vi "VI Tree.vi"   [LabVIEW 2014, in "Newport ESP301.lvlib"]
doc: "This is the instrument driver for the <INSTRUMENT NAME>. The VI Tree displays all the user-callable VIs of the instrument driver in an organized table.\n\nNOTE :\nEvery VIs need the VISA Ressource Name parameter for working."
uses:
  Newport ESP301.lvlib
panel:
  # "(c) 2009 <Newport>.  ALL RIGHTS RESERVED."
  # "SEE DIAGRAM\nFOR VI TREE."
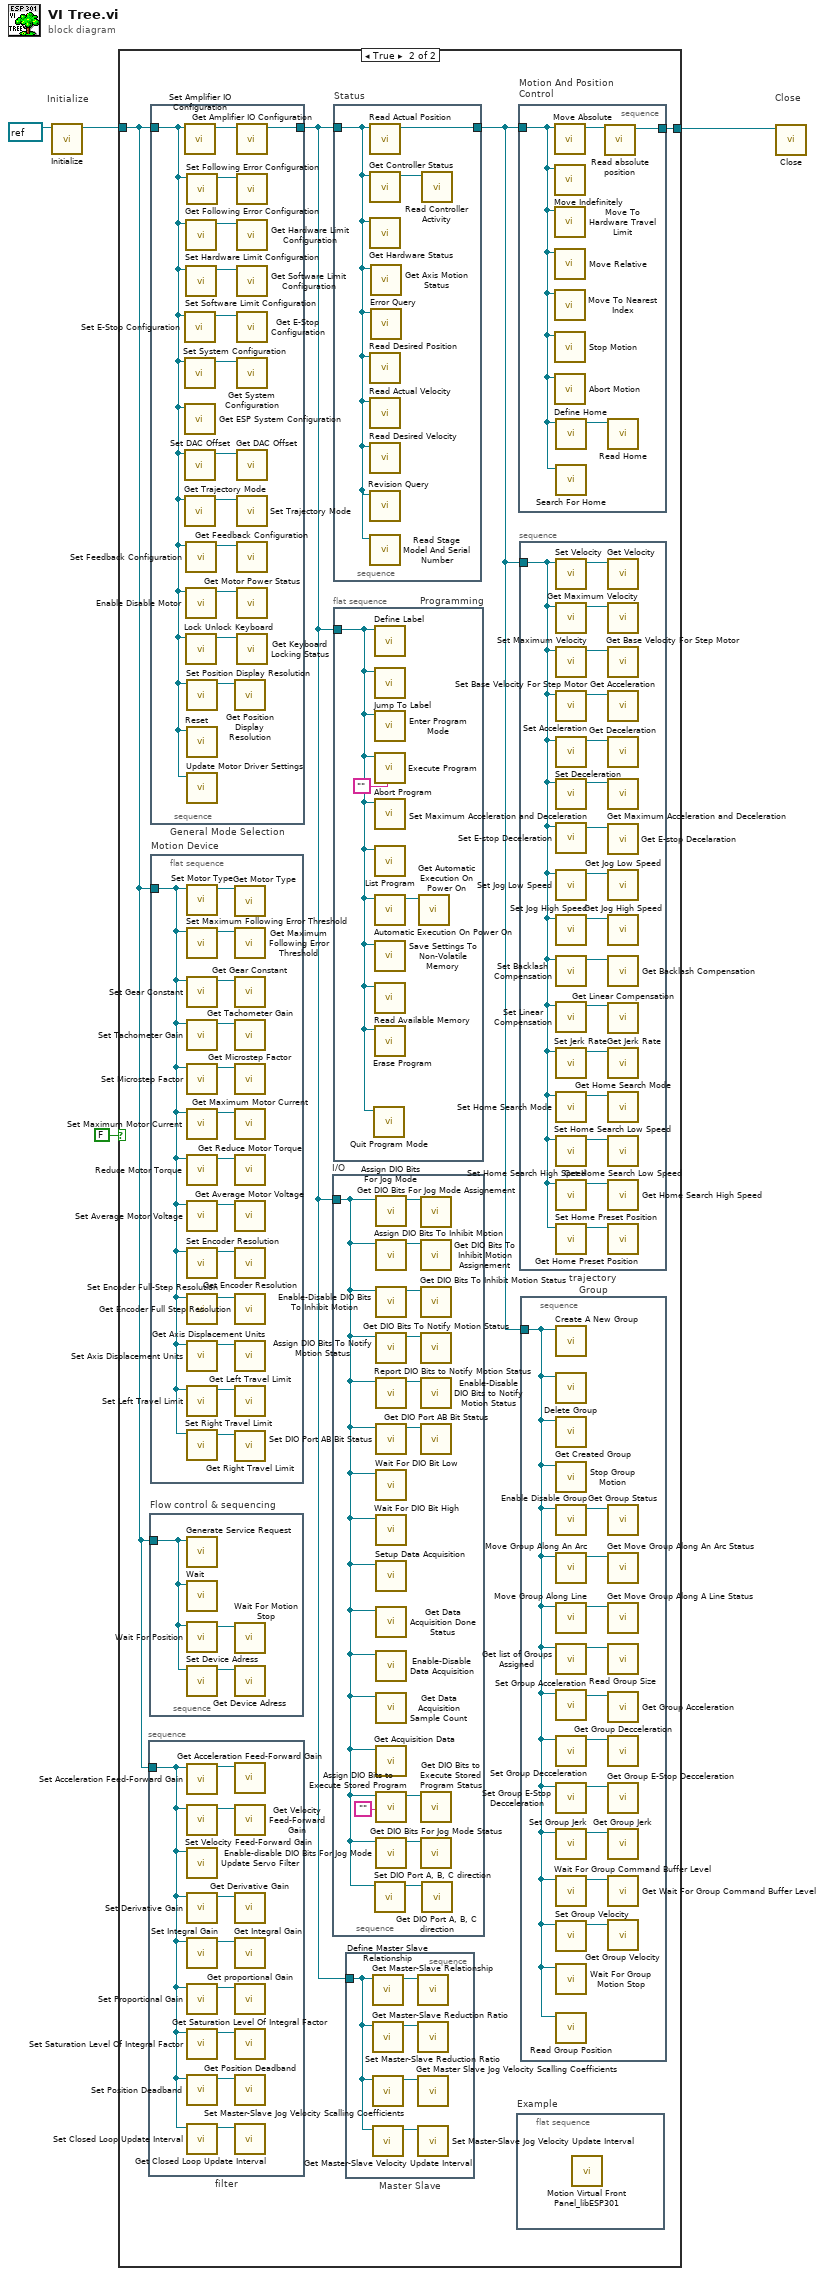
[diagram p0: block diagram]
diagram:
  # "Close"
  # "Initialize"
  n1 = call "Initialize.vi"("VISA resource name"=refnum<visa-resource-name> refnum) -> ("VISA resource name out"=w3:refnum<visa-resource-name>)  [unwired: 8 in, 1 out]
  n2 = case shown="True" FALSE {
    tunnel: w3 -> [w5 w8]
    tunnel: [w5 w6] -> w2
    frame False {
    }
    frame True {
      n3 = stacked-sequence "filter" {
        tunnel: w8 -> [w65]
        frame #0 {
          n4 = call "Set Acceleration Feed-Forward Gain.vi"("VISA resource name"=w65) -> ("VISA resource name out"=w66:refnum<visa-resource-name>)  [unwired: 5 in, 1 out]
          n5 = call "Set Velocity Feed-Forward Gain.vi"("VISA resource name"=w65) -> ("VISA resource name out"=w67:refnum<visa-resource-name>)  [unwired: 5 in, 1 out]
          n6 = call "Update Servo Filter.vi"("VISA resource name"=w65) -> ()  [unwired: 5 in, 2 out]
          n7 = call "Set Derivative Gain.vi"("VISA resource name"=w65) -> ("VISA resource name out"=w71:refnum<visa-resource-name>)  [unwired: 5 in, 1 out]
          n8 = call "Set Integral Gain.vi"("VISA resource name"=w65) -> ("VISA resource name out"=w72:refnum<visa-resource-name>)  [unwired: 5 in, 1 out]
          n9 = call "Set Proportional Gain.vi"("VISA resource name"=w65) -> ("VISA resource name out"=w70:refnum<visa-resource-name>)  [unwired: 5 in, 1 out]
          n10 = call "Set Saturation Level Of Integral Factor.vi"("VISA resource name"=w65) -> ("VISA resource name out"=w69:refnum<visa-resource-name>)  [unwired: 5 in, 1 out]
          n11 = call "Set Position Deadband.vi"("VISA resource name"=w65) -> ("VISA resource name out"=w68:refnum<visa-resource-name>)  [unwired: 5 in, 1 out]
          n12 = call "Set Closed Loop Update Interval.vi"("VISA resource name"=w65) -> ("VISA resource name out"=w64:refnum<visa-resource-name>)  [unwired: 5 in, 1 out]
          n13 = call "Get Acceleration Feed-Forward Gain.vi"("VISA resource name"=w66) -> ()  [unwired: 4 in, 3 out]
          n14 = call "Get Velocity Feed-Forward Gain.vi"("VISA resource name"=w67) -> ()  [unwired: 4 in, 3 out]
          n15 = call "Get Derivative Gain.vi"("VISA resource name"=w71) -> ()  [unwired: 4 in, 3 out]
          n16 = call "Get Integral Gain.vi"("VISA resource name"=w72) -> ()  [unwired: 4 in, 3 out]
          n17 = call "Get proportional Gain.vi"("VISA resource name"=w70) -> ()  [unwired: 4 in, 3 out]
          n18 = call "Get Saturation Level Of Integral Factor.vi"("VISA resource name"=w69) -> ()  [unwired: 4 in, 3 out]
          n19 = call "Get Position Deadband.vi"("VISA resource name"=w68) -> ()  [unwired: 4 in, 3 out]
          n20 = call "Get Closed Loop Update Interval.vi"("VISA resource name"=w64) -> ()  [unwired: 4 in, 3 out]
        }
      }
      n21 = stacked-sequence "Flow control & sequencing" {
        tunnel: w8 -> [w36]
        frame #0 {
          n22 = call "Generate Service Request.vi"("VISA resource name"=w36) -> ()  [unwired: 5 in, 2 out]
          n23 = call "Wait.vi"("VISA resource name"=w36) -> ()  [unwired: 5 in, 2 out]
          n24 = call "Wait For Position.vi"("VISA resource name"=w36) -> ("VISA resource name out"=w38:refnum<visa-resource-name>)  [unwired: 5 in, 1 out]
          n25 = call "Set Device Adress.vi"("VISA resource name"=w36) -> ("VISA resource name out"=w37:refnum<visa-resource-name>)  [unwired: 5 in, 1 out]
          n26 = call "Wait For Motion Stop.vi"("VISA resource name"=w38) -> ()  [unwired: 5 in, 2 out]
          n27 = call "Get Device Adress.vi"("VISA resource name"=w37) -> ()  [unwired: 4 in, 3 out]
        }
      }
      n28 = stacked-sequence "General Mode Selection" {
        tunnel: w8 -> [w23]
        tunnel: [w22] -> w7
        frame #0 {
          n29 = call "Set Amplifier IO Configuration.vi"("VISA resource name"=w23) -> ("VISA resource name out"=w31:refnum<visa-resource-name>)  [unwired: 5 in, 1 out]
          n30 = call "Set E-Stop Configuration.vi"("VISA resource name"=w23) -> ("VISA resource name out"=w32:refnum<visa-resource-name>)  [unwired: 5 in, 1 out]
          n31 = call "Set System Configuration.vi"("VISA resource name"=w23) -> ("VISA resource name out"=w28:refnum<visa-resource-name>)  [unwired: 5 in, 1 out]
          n32 = call "Get ESP System Configuration.vi"("VISA resource name"=w23) -> ()  [unwired: 4 in, 3 out]
          n33 = call "Set DAC Offset.vi"("VISA resource name"=w23) -> ("VISA resource name out"=w30:refnum<visa-resource-name>)  [unwired: 5 in, 1 out]
          n34 = call "Get Trajectory Mode.vi"("VISA resource name"=w23) -> ("VISA resource name out"=w29:refnum<visa-resource-name>)  [unwired: 4 in, 2 out]
          n35 = call "Set Hardware Limit Configuration.vi"("VISA resource name"=w23) -> ("VISA resource name out"=w35:refnum<visa-resource-name>)  [unwired: 5 in, 1 out]
          n36 = call "Set Software Limit Configuration.vi"("VISA resource name"=w23) -> ("VISA resource name out"=w33:refnum<visa-resource-name>)  [unwired: 5 in, 1 out]
          n37 = call "Set Feedback Configuration.vi"("VISA resource name"=w23) -> ("VISA resource name out"=w27:refnum<visa-resource-name>)  [unwired: 5 in, 1 out]
          n38 = call "Enable Disable Motor.vi"("VISA resource name"=w23) -> ("VISA resource name out"=w26:refnum<visa-resource-name>)  [unwired: 5 in, 1 out]
          n39 = call "Lock Unlock Keyboard.vi"("VISA resource name"=w23) -> ("VISA resource name out"=w25:refnum<visa-resource-name>)  [unwired: 5 in, 1 out]
          n40 = call "Set Following Error Configuration.vi"("VISA resource name"=w23) -> ("VISA resource name out"=w34:refnum<visa-resource-name>)  [unwired: 5 in, 1 out]
          n41 = call "Set Position Display Resolution.vi"("VISA resource name"=w23) -> ("VISA resource name out"=w24:refnum<visa-resource-name>)  [unwired: 5 in, 1 out]
          n42 = call "Reset.vi"("VISA resource name"=w23) -> ()  [unwired: 5 in, 2 out]
          n43 = call "Update Motor Driver Settings.vi"("VISA resource name"=w23) -> ()  [unwired: 5 in, 2 out]
          n44 = call "Get Position Display Resolution.vi"("VISA resource name"=w24) -> ()  [unwired: 4 in, 3 out]
          n45 = call "Get Amplifier IO Configuration.vi"("VISA resource name"=w31) -> ("VISA resource name out"=w22:refnum<visa-resource-name>)  [unwired: 4 in, 2 out]
          n46 = call "Get Following Error Configuration.vi"("VISA resource name"=w34) -> ()  [unwired: 4 in, 3 out]
          n47 = call "Get Hardware Limit Configuration.vi"("VISA resource name"=w35) -> ()  [unwired: 4 in, 3 out]
          n48 = call "Get Software Limit Configuration.vi"("VISA resource name"=w33) -> ()  [unwired: 4 in, 3 out]
          n49 = call "Get E-Stop Configuration.vi"("VISA resource name"=w32) -> ()  [unwired: 4 in, 3 out]
          n50 = call "Get System Configuration.vi"("VISA resource name"=w28) -> ()  [unwired: 4 in, 3 out]
          n51 = call "Get DAC Offset.vi"("VISA resource name"=w30) -> ()  [unwired: 4 in, 3 out]
          n52 = call "Set Trajectory Mode.vi"("VISA resource name"=w29) -> ()  [unwired: 6 in, 2 out]
          n53 = call "Get Feedback Configuration.vi"("VISA resource name"=w27) -> ()  [unwired: 4 in, 3 out]
          n54 = call "Get Motor Power Status.vi"("VISA resource name"=w26) -> ()  [unwired: 4 in, 3 out]
          n55 = call "Get Keyboard Locking Status.vi"("VISA resource name"=w25) -> ()  [unwired: 4 in, 3 out]
        }
      }
      n56 = flat-sequence "Motion Device" {
        tunnel: w8 -> [w91]
        frame #0 {
          n57 = call "Set Motor Type.vi"("VISA resource name"=w91) -> ("VISA resource name out"=w103:refnum<visa-resource-name>)  [unwired: 6 in, 1 out]
          n58 = call "Set Maximum Following Error Threshold.vi"("VISA resource name"=w91) -> ("VISA resource name out"=w102:refnum<visa-resource-name>)  [unwired: 5 in, 1 out]
          n59 = call "Set Gear Constant.vi"("VISA resource name"=w91) -> ("VISA resource name out"=w99:refnum<visa-resource-name>)  [unwired: 5 in, 1 out]
          n60 = call "Set Tachometer Gain.vi"("VISA resource name"=w91) -> ("VISA resource name out"=w101:refnum<visa-resource-name>)  [unwired: 5 in, 1 out]
          n61 = call "Set Microstep Factor.vi"("VISA resource name"=w91) -> ("VISA resource name out"=w100:refnum<visa-resource-name>)  [unwired: 5 in, 1 out]
          n62 = call "Set Maximum Motor Current.vi"("VISA resource name"=w91) -> ("VISA resource name out"=w90:refnum<visa-resource-name>)  [unwired: 5 in, 1 out]
          n63 = call "Reduce Motor Torque.vi"("VISA resource name"=w91) -> ("VISA resource name out"=w98:refnum<visa-resource-name>)  [unwired: 6 in, 1 out]
          n64 = call "Set Average Motor Voltage.vi"("VISA resource name"=w91) -> ("VISA resource name out"=w97:refnum<visa-resource-name>)  [unwired: 5 in, 1 out]
          n65 = call "Set Encoder Resolution.vi"("VISA resource name"=w91) -> ("VISA resource name out"=w96:refnum<visa-resource-name>)  [unwired: 5 in, 1 out]
          n66 = call "Set Encoder Full-Step Resolution.vi"("VISA resource name"=w91) -> ("VISA resource name out"=w95:refnum<visa-resource-name>)  [unwired: 5 in, 1 out]
          n67 = call "Set Axis Displacement Units.vi"("VISA resource name"=w91) -> ("VISA resource name out"=w92:refnum<visa-resource-name>)  [unwired: 6 in, 1 out]
          n68 = call "Set Left Travel Limit.vi"("VISA resource name"=w91) -> ("VISA resource name out"=w94:refnum<visa-resource-name>)  [unwired: 5 in, 1 out]
          n69 = call "Set Right Travel Limit.vi"("VISA resource name"=w91) -> ("VISA resource name out"=w93:refnum<visa-resource-name>)  [unwired: 5 in, 1 out]
          n70 = call "Get Motor Type.vi"("VISA resource name"=w103) -> ()  [unwired: 4 in, 3 out]
          n71 = call "Get Maximum Following Error Threshold.vi"("VISA resource name"=w102) -> ()  [unwired: 4 in, 3 out]
          n72 = call "Get Gear Constant.vi"("VISA resource name"=w99) -> ()  [unwired: 4 in, 3 out]
          n73 = call "Get Tachometer Gain.vi"("VISA resource name"=w101) -> ()  [unwired: 4 in, 3 out]
          n74 = call "Get Microstep Factor.vi"("VISA resource name"=w100) -> ()  [unwired: 4 in, 3 out]
          n75 = call "Get Maximum Motor Current.vi"("VISA resource name"=w90) -> ()  [unwired: 4 in, 3 out]
          n76 = call "Get Reduce Motor Torque.vi"("VISA resource name"=w98) -> ()  [unwired: 4 in, 3 out]
          n77 = call "Get Average Motor Voltage.vi"("VISA resource name"=w97) -> ()  [unwired: 4 in, 3 out]
          n78 = call "Get Encoder Resolution.vi"("VISA resource name"=w96) -> ()  [unwired: 4 in, 3 out]
          n79 = call "Get Encoder Full Step Resolution.vi"("VISA resource name"=w95) -> ()  [unwired: 4 in, 3 out]
          n80 = call "Get Axis Displacement Units.vi"("VISA resource name"=w92) -> ()  [unwired: 4 in, 3 out]
          n81 = call "Get Left Travel Limit.vi"("VISA resource name"=w94) -> ()  [unwired: 4 in, 3 out]
          n82 = call "Get Right Travel Limit.vi"("VISA resource name"=w93) -> ()  [unwired: 4 in, 3 out]
        }
      }
      n83 = stacked-sequence "I/O" {
        tunnel: w7 -> [w42]
        frame #0 {
          n84 = call "Set DIO Port A, B, C direction.vi"("VISA resource name"=w42) -> ("VISA resource name out"=w43:refnum<visa-resource-name>)  [unwired: 9 in, 1 out]
          n85 = call "Assign DIO Bits For Jog Mode.vi"("VISA resource name"=w42) -> ("VISA resource name out"=w52:refnum<visa-resource-name>)  [unwired: 6 in, 1 out]
          n86 = call "Assign DIO Bits To Inhibit Motion.vi"("VISA resource name"=w42) -> ("VISA resource name out"=w47:refnum<visa-resource-name>)  [unwired: 6 in, 1 out]
          n87 = call "Enable-Disable DIO Bits To Inhibit Motion.vi"("VISA resource name"=w42) -> ("VISA resource name out"=w48:refnum<visa-resource-name>)  [unwired: 5 in, 1 out]
          n88 = call "Assign DIO Bits To Notify Motion Status.vi"("VISA resource name"=w42) -> ("VISA resource name out"=w49:refnum<visa-resource-name>)  [unwired: 6 in, 1 out]
          n89 = call "Report DIO Bits to Notify Motion Status.vi"("VISA resource name"=w42) -> ("VISA resource name out"=w51:refnum<visa-resource-name>)  [unwired: 4 in, 2 out]
          n90 = call "Set DIO Port AB Bit Status.vi"("VISA resource name"=w42) -> ("VISA resource name out"=w50:refnum<visa-resource-name>)  [unwired: 5 in, 1 out]
          n91 = call "Wait For DIO Bit Low.vi"("VISA resource name"=w42) -> ()  [unwired: 5 in, 2 out]
          n92 = call "Wait For DIO Bit High.vi"("VISA resource name"=w42) -> ()  [unwired: 5 in, 2 out]
          n93 = call "Setup Data Acquisition.vi"("VISA resource name"=w42) -> ()  [unwired: 5 in, 2 out]
          n94 = call "Get Data Acquisition Done Status.vi"("VISA resource name"=w42) -> ()  [unwired: 4 in, 3 out]
          n95 = call "Enable-Disable Data Acquisition.vi"("VISA resource name"=w42) -> ()  [unwired: 5 in, 2 out]
          n96 = call "Get Data Acquisition Sample Count.vi"("VISA resource name"=w42) -> ()  [unwired: 4 in, 3 out]
          n97 = call "Get Acquisition Data.vi"("VISA resource name"=w42) -> ()  [unwired: 4 in, 3 out]
          n98 = call "Assign DIO Bits to Execute Stored Program.vi"("Program Name"="", "VISA resource name"=w42) -> ("VISA resource name out"=w46:refnum<visa-resource-name>)  [unwired: 4 in, 1 out]
          n99 = call "Enable-disable DIO Bits For Jog Mode.vi"("VISA resource name"=w42) -> ("VISA resource name out"=w44:refnum<visa-resource-name>)  [unwired: 5 in, 1 out]
          n100 = call "Get DIO Bits For Jog Mode Assignement.vi"("VISA resource name"=w52) -> ()  [unwired: 3 in, 4 out]
          n101 = call "Get DIO Bits To Inhibit Motion Assignement.vi"("VISA resource name"=w47) -> ()  [unwired: 3 in, 4 out]
          n102 = call "Get DIO Bits To Inhibit Motion Status.vi"("VISA resource name"=w48) -> ()  [unwired: 4 in, 3 out]
          n103 = call "Get DIO Bits To Notify Motion Status.vi"("VISA resource name"=w49) -> ()  [unwired: 3 in, 4 out]
          n104 = call "Enable-Disable DIO Bits to Notify Motion Status.vi"("VISA resource name"=w51) -> ()  [unwired: 5 in, 2 out]
          n105 = call "Get DIO Port AB Bit Status.vi"("VISA resource name"=w50) -> ()  [unwired: 4 in, 3 out]
          n106 = call "Get DIO Bits to Execute Stored Program Status.vi"("VISA resource name"=w46) -> ()  [unwired: 4 in, 3 out]
          n107 = call "Get DIO Bits For Jog Mode Status.vi"("VISA resource name"=w44) -> ()  [unwired: 4 in, 3 out]
          n108 = call "Get DIO Port A, B, C direction.vi"("VISA resource name"=w43) -> ()  [unwired: 8 in, 3 out]
        }
      }
      n109 = stacked-sequence "Status" {
        tunnel: w7 -> [w15]
        tunnel: [w14] -> w9
        frame #0 {
          n110 = call "Read Actual Position.vi"("VISA resource name"=w15) -> ("VISA resource name out"=w14:refnum<visa-resource-name>)  [unwired: 4 in, 2 out]
          n111 = call "Get Controller Status.vi"("VISA resource name"=w15) -> ("VISA resource name out"=w16:refnum<visa-resource-name>)  [unwired: 3 in, 3 out]
          n112 = call "Get Hardware Status.vi"("VISA resource name"=w15) -> ()  [unwired: 3 in, 4 out]
          n113 = call "Read Desired Position.vi"("VISA resource name"=w15) -> ()  [unwired: 4 in, 3 out]
          n114 = call "Read Actual Velocity.vi"("VISA resource name"=w15) -> ()  [unwired: 4 in, 3 out]
          n115 = call "Read Desired Velocity.vi"("VISA resource name"=w15) -> ()  [unwired: 4 in, 3 out]
          n116 = call "Revision Query.vi"("VISA resource name"=w15) -> ()  [unwired: 7 in, 4 out]
          n117 = call "Read Stage Model And Serial Number.vi"("VISA resource name"=w15) -> ()  [unwired: 3 in, 4 out]
          n118 = call "Get Axis Motion Status.vi"("VISA resource name"=w15) -> ()  [unwired: 4 in, 3 out]
          n119 = call "Error Query.vi"("VISA resource name"=w15) -> ()  [unwired: 3 in, 4 out]
          n120 = call "Read Controller Activity.vi"("VISA resource name"=w16) -> ()  [unwired: 4 in, 3 out]
        }
      }
      n121 = flat-sequence "Programming" {
        tunnel: w7 -> [w39]
        frame #0 {
          n122 = call "Quit Program Mode.vi"("VISA resource name"=w39) -> ()  [unwired: 5 in, 2 out]
          n123 = call "Define Label.vi"("VISA resource name"=w39) -> ()  [unwired: 5 in, 2 out]
          n124 = call "Jump To Label.vi"("VISA resource name"=w39) -> ()  [unwired: 5 in, 2 out]
          n125 = call "Enter Program Mode.vi"("VISA resource name"=w39) -> ()  [unwired: 5 in, 2 out]
          n126 = call "Execute Program.vi"("Program Name"="", "VISA resource name"=w39) -> ()  [unwired: 4 in, 2 out]
          n127 = call "Abort Program.vi"("VISA resource name"=w39) -> ()  [unwired: 5 in, 2 out]
          n128 = call "List Program.vi"("VISA resource name"=w39) -> ()  [unwired: 4 in, 3 out]
          n129 = call "Automatic Execution On Power On.vi"("VISA resource name"=w39) -> ("VISA resource name out"=w40:refnum<visa-resource-name>)  [unwired: 5 in, 1 out]
          n130 = call "Save Settings To Non-Volatile Memory.vi"("VISA resource name"=w39) -> ()  [unwired: 5 in, 2 out]
          n131 = call "Read Available Memory.vi"("VISA resource name"=w39) -> ()  [unwired: 5 in, 2 out]
          n132 = call "Erase Program.vi"("VISA resource name"=w39) -> ()  [unwired: 5 in, 2 out]
          n133 = call "Get Automatic Execution On Power On.vi"("VISA resource name"=w40) -> ()  [unwired: 3 in, 4 out]
        }
      }
      n134 = stacked-sequence "Master Slave" {
        tunnel: w7 -> [w17]
        frame #0 {
          n135 = call "Define Master Slave Relationship.vi"("VISA resource name"=w17) -> ("VISA resource name out"=w21:refnum<visa-resource-name>)  [unwired: 5 in, 1 out]
          n136 = call "Get Master-Slave Reduction Ratio.vi"("VISA resource name"=w17) -> ("VISA resource name out"=w20:refnum<visa-resource-name>)  [unwired: 4 in, 2 out]
          n137 = call "Set Master-Slave Jog Velocity Scalling Coefficients.vi"("VISA resource name"=w17) -> ("VISA resource name out"=w18:refnum<visa-resource-name>)  [unwired: 5 in, 1 out]
          n138 = call "Get Master-Slave Velocity Update Interval.vi"("VISA resource name"=w17) -> ("VISA resource name out"=w19:refnum<visa-resource-name>)  [unwired: 4 in, 2 out]
          n139 = call "Get Master-Slave Relationship.vi"("VISA resource name"=w21) -> ()  [unwired: 4 in, 3 out]
          n140 = call "Set Master-Slave Reduction Ratio.vi"("VISA resource name"=w20) -> ()  [unwired: 5 in, 2 out]
          n141 = call "Get Master Slave Jog Velocity Scalling Coefficients.vi"("VISA resource name"=w18) -> ()  [unwired: 3 in, 4 out]
          n142 = call "Set Master-Slave Jog Velocity Update Interval.vi"("VISA resource name"=w19) -> ()  [unwired: 5 in, 2 out]
        }
      }
      n143 = flat-sequence "Example" {
        frame #0 {
          n144 = call "Motion Virtual Front Panel_libESP301.vi"() -> ()  [unwired: 1 in]
        }
      }
      n145 = stacked-sequence "Motion And Position \nControl" {
        tunnel: w9 -> [w12]
        tunnel: [w10] -> w6
        frame #0 {
          n146 = call "Move Absolute.vi"("VISA resource name"=w12) -> ("VISA resource name out"=w13:refnum<visa-resource-name>)  [unwired: 5 in, 1 out]
          n147 = call "Move Indefinitely.vi"("VISA resource name"=w12) -> ()  [unwired: 5 in, 2 out]
          n148 = call "Move To Hardware Travel Limit.vi"("VISA resource name"=w12) -> ()  [unwired: 5 in, 2 out]
          n149 = call "Move Relative.vi"("VISA resource name"=w12) -> ()  [unwired: 5 in, 2 out]
          n150 = call "Move To Nearest Index.vi"("VISA resource name"=w12) -> ()  [unwired: 5 in, 2 out]
          n151 = call "Stop Motion.vi"("VISA resource name"=w12) -> ()  [unwired: 5 in, 2 out]
          n152 = call "Abort Motion.vi"("VISA resource name"=w12) -> ()  [unwired: 5 in, 2 out]
          n153 = call "Define Home.vi"("VISA resource name"=w12) -> ("VISA resource name out"=w11:refnum<visa-resource-name>)  [unwired: 5 in, 1 out]
          n154 = call "Search For Home.vi"("VISA resource name"=w12) -> ()  [unwired: 6 in, 2 out]
          n155 = call "Read absolute position.vi"("VISA resource name"=w13) -> ("VISA resource name out"=w10:refnum<visa-resource-name>)  [unwired: 4 in, 2 out]
          n156 = call "Read Home.vi"("VISA resource name"=w11) -> ()  [unwired: 4 in, 3 out]
        }
      }
      n157 = stacked-sequence "trajectory" {
        tunnel: w9 -> [w73]
        frame #0 {
          n158 = call "Set Velocity.vi"("VISA resource name"=w73) -> ("VISA resource name out"=w89:refnum<visa-resource-name>)  [unwired: 5 in, 1 out]
          n159 = call "Set Maximum Velocity.vi"("VISA resource name"=w73) -> ("VISA resource name out"=w88:refnum<visa-resource-name>)  [unwired: 5 in, 1 out]
          n160 = call "Set Base Velocity For Step Motor.vi"("VISA resource name"=w73) -> ("VISA resource name out"=w87:refnum<visa-resource-name>)  [unwired: 5 in, 1 out]
          n161 = call "Set Acceleration.vi"("VISA resource name"=w73) -> ("VISA resource name out"=w85:refnum<visa-resource-name>)  [unwired: 5 in, 1 out]
          n162 = call "Set Deceleration.vi"("VISA resource name"=w73) -> ("VISA resource name out"=w86:refnum<visa-resource-name>)  [unwired: 5 in, 1 out]
          n163 = call "Set Maximum Acceleration and Deceleration.vi"("VISA resource name"=w73) -> ("VISA resource name out"=w84:refnum<visa-resource-name>)  [unwired: 5 in, 1 out]
          n164 = call "Set E-stop Deceleration.vi"("VISA resource name"=w73) -> ("VISA resource name out"=w83:refnum<visa-resource-name>)  [unwired: 5 in, 1 out]
          n165 = call "Set Jog Low Speed.vi"("VISA resource name"=w73) -> ("VISA resource name out"=w81:refnum<visa-resource-name>)  [unwired: 5 in, 1 out]
          n166 = call "Set Jog High Speed.vi"("VISA resource name"=w73) -> ("VISA resource name out"=w80:refnum<visa-resource-name>)  [unwired: 5 in, 1 out]
          n167 = call "Set Backlash Compensation.vi"("VISA resource name"=w73) -> ("VISA resource name out"=w82:refnum<visa-resource-name>)  [unwired: 5 in, 1 out]
          n168 = call "Set Linear Compensation.vi"("VISA resource name"=w73) -> ("VISA resource name out"=w78:refnum<visa-resource-name>)  [unwired: 5 in, 1 out]
          n169 = call "Set Jerk Rate.vi"("VISA resource name"=w73) -> ("VISA resource name out"=w79:refnum<visa-resource-name>)  [unwired: 5 in, 1 out]
          n170 = call "Set Home Search Mode.vi"("VISA resource name"=w73) -> ("VISA resource name out"=w74:refnum<visa-resource-name>)  [unwired: 6 in, 1 out]
          n171 = call "Set Home Search Low Speed.vi"("VISA resource name"=w73) -> ("VISA resource name out"=w75:refnum<visa-resource-name>)  [unwired: 5 in, 1 out]
          n172 = call "Set Home Search High Speed.vi"("VISA resource name"=w73) -> ("VISA resource name out"=w76:refnum<visa-resource-name>)  [unwired: 5 in, 1 out]
          n173 = call "Set Home Preset Position.vi"("VISA resource name"=w73) -> ("VISA resource name out"=w77:refnum<visa-resource-name>)  [unwired: 5 in, 1 out]
          n174 = call "Get Velocity.vi"("VISA resource name"=w89) -> ()  [unwired: 4 in, 3 out]
          n175 = call "Get Maximum Velocity.vi"("VISA resource name"=w88) -> ()  [unwired: 4 in, 3 out]
          n176 = call "Get Base Velocity For Step Motor.vi"("VISA resource name"=w87) -> ()  [unwired: 4 in, 3 out]
          n177 = call "Get Acceleration.vi"("VISA resource name"=w85) -> ()  [unwired: 4 in, 3 out]
          n178 = call "Get Deceleration.vi"("VISA resource name"=w86) -> ()  [unwired: 4 in, 3 out]
          n179 = call "Get Maximum Acceleration and Deceleration.vi"("VISA resource name"=w84) -> ()  [unwired: 4 in, 3 out]
          n180 = call "Get E-stop Decelaration.vi"("VISA resource name"=w83) -> ()  [unwired: 4 in, 3 out]
          n181 = call "Get Jog Low Speed.vi"("VISA resource name"=w81) -> ()  [unwired: 4 in, 3 out]
          n182 = call "Get Jog High Speed.vi"("VISA resource name"=w80) -> ()  [unwired: 4 in, 3 out]
          n183 = call "Get Backlash Compensation.vi"("VISA resource name"=w82) -> ()  [unwired: 4 in, 3 out]
          n184 = call "Get Linear Compensation.vi"("VISA resource name"=w78) -> ()  [unwired: 4 in, 3 out]
          n185 = call "Get Jerk Rate.vi"("VISA resource name"=w79) -> ()  [unwired: 4 in, 3 out]
          n186 = call "Get Home Search Mode.vi"("VISA resource name"=w74) -> ()  [unwired: 4 in, 3 out]
          n187 = call "Get Home Search Low Speed.vi"("VISA resource name"=w75) -> ()  [unwired: 4 in, 3 out]
          n188 = call "Get Home Search High Speed.vi"("VISA resource name"=w76) -> ()  [unwired: 4 in, 3 out]
          n189 = call "Get Home Preset Position.vi"("VISA resource name"=w77) -> ()  [unwired: 4 in, 3 out]
        }
      }
      n190 = stacked-sequence "Group" {
        tunnel: w9 -> [w53]
        frame #0 {
          n191 = call "Create A New Group.vi"("VISA resource name"=w53) -> ()  [unwired: 5 in, 2 out]
          n192 = call "Delete Group.vi"("VISA resource name"=w53) -> ()  [unwired: 5 in, 2 out]
          n193 = call "Get Created Group.vi"("VISA resource name"=w53) -> ()  [unwired: 4 in, 3 out]
          n194 = call "Stop Group Motion.vi"("VISA resource name"=w53) -> ()  [unwired: 5 in, 2 out]
          n195 = call "Enable Disable Group.vi"("VISA resource name"=w53) -> ("VISA resource name out"=w56:refnum<visa-resource-name>)  [unwired: 5 in, 1 out]
          n196 = call "Move Group Along An Arc.vi"("VISA resource name"=w53) -> ("VISA resource name out"=w54:refnum<visa-resource-name>)  [unwired: 5 in, 1 out]
          n197 = call "Move Group Along Line.vi"("VISA resource name"=w53) -> ("VISA resource name out"=w55:refnum<visa-resource-name>)  [unwired: 5 in, 1 out]
          n198 = call "Get list of Groups Assigned.vi"("VISA resource name"=w53) -> ("VISA resource name out"=w63:refnum<visa-resource-name>)  [unwired: 4 in, 2 out]
          n199 = call "Set Group Acceleration.vi"("VISA resource name"=w53) -> ("VISA resource name out"=w62:refnum<visa-resource-name>)  [unwired: 5 in, 1 out]
          n200 = call "Set Group Decceleration.vi"("VISA resource name"=w53) -> ("VISA resource name out"=w61:refnum<visa-resource-name>)  [unwired: 5 in, 1 out]
          n201 = call "Set Group E-Stop Decceleration.vi"("VISA resource name"=w53) -> ("VISA resource name out"=w60:refnum<visa-resource-name>)  [unwired: 5 in, 1 out]
          n202 = call "Set Group Jerk.vi"("VISA resource name"=w53) -> ("VISA resource name out"=w59:refnum<visa-resource-name>)  [unwired: 5 in, 1 out]
          n203 = call "Wait For Group Command Buffer Level.vi"("VISA resource name"=w53) -> ("VISA resource name out"=w58:refnum<visa-resource-name>)  [unwired: 5 in, 1 out]
          n204 = call "Set Group Velocity.vi"("VISA resource name"=w53) -> ("VISA resource name out"=w57:refnum<visa-resource-name>)  [unwired: 5 in, 1 out]
          n205 = call "Wait For Group Motion Stop.vi"("VISA resource name"=w53) -> ()  [unwired: 5 in, 2 out]
          n206 = call "Read Group Position.vi"("VISA resource name"=w53) -> ()  [unwired: 4 in, 3 out]
          n207 = call "Get Group Status.vi"("VISA resource name"=w56) -> ()  [unwired: 4 in, 3 out]
          n208 = call "Get Move Group Along An Arc Status.vi"("VISA resource name"=w54) -> ()  [unwired: 4 in, 3 out]
          n209 = call "Get Move Group Along A Line Status.vi"("VISA resource name"=w55) -> ()  [unwired: 4 in, 3 out]
          n210 = call "Read Group Size.vi"("VISA resource name"=w63) -> ()  [unwired: 4 in, 3 out]
          n211 = call "Get Group Acceleration.vi"("VISA resource name"=w62) -> ()  [unwired: 4 in, 3 out]
          n212 = call "Get Group Decceleration.vi"("VISA resource name"=w61) -> ()  [unwired: 4 in, 3 out]
          n213 = call "Get Group E-Stop Decceleration.vi"("VISA resource name"=w60) -> ()  [unwired: 4 in, 3 out]
          n214 = call "Get Group Jerk.vi"("VISA resource name"=w59) -> ()  [unwired: 4 in, 3 out]
          n215 = call "Get Wait For Group Command Buffer Level.vi"("VISA resource name"=w58) -> ()  [unwired: 4 in, 3 out]
          n216 = call "Get Group Velocity.vi"("VISA resource name"=w57) -> ()  [unwired: 4 in, 3 out]
        }
      }
    }
  }
  n217 = call "Close.vi"("VISA resource name"=w2) -> ()  [unwired: 10 in, 1 out]
